vi "Set Value State on Multiple Controls.vi"(10 "Value":bool, 11 "Controls":refnum<vi>[](array[refnum])) -> ()   [LabVIEW 2015]
doc: "Sets all the controls in the input array to the \"Enable state\" value."
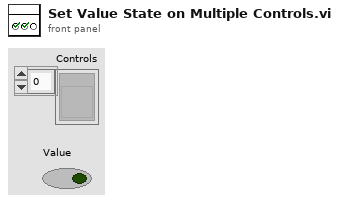
[diagram p1: front panel]
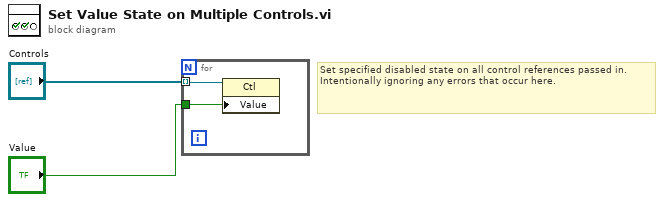
[diagram p0: block diagram]
diagram:
  # "Set specified disabled state on all control references passed in. Intentionally ignoring any errors that occur here."
  n1 = for {
    tunnel: "Controls" -> [w4] mode=indexing
    tunnel: "Value" -> [w3]
    n2 = property class="Ctl"(reference=w4, "Value"=w3) -> ()  [unwired: 1 in, 2 out]
  }
